vi "CAENHV Get Ch Param Prop String.vi"(6 "PropName":string, 7 "ParName":string, 8 "error in (no error)":errorcluster, 9 "Ch":u16, 10 "slot":u16, 11 "handle":i32) -> (0 "error out":errorcluster, 3 "retval":string)   [LabVIEW 2009, in "CAENHVWrapper.lvlib"]
doc: "CAENHVLIB_API CAENHVRESULT CAENHV_GetChParamProp(int handle, \n ushort slot, ushort Ch, const char *ParName, const char *PropName, void *retval);"
uses:
  <userlib>/CAENHVWrapper/CAENHVWrapper.lvlib
  <userlib>/CAENHVWrapper/CAENHVWrapper.dll
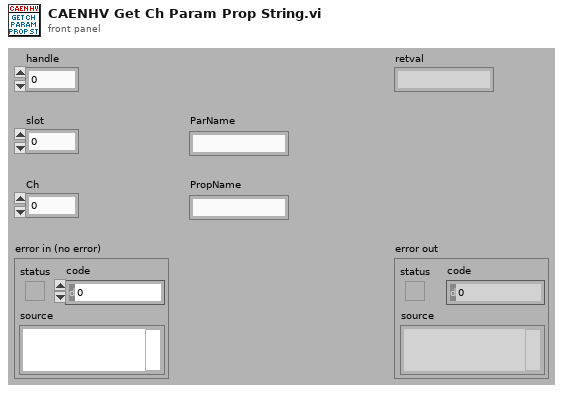
[diagram p1: front panel]
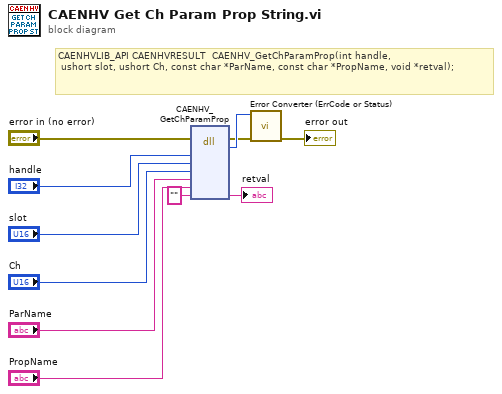
[diagram p0: block diagram]
diagram:
  # "CAENHVLIB_API CAENHVRESULT  CAENHV_GetChParamProp(int handle, \n ushort slot, ushort Ch, const char *ParName, const char *PropName, void *retval);"
  n1 = dll-call lib="C:/Program Files/National Instruments/LabVIEW 2009/user.lib/CAENHVWrapper/CAENHVWrapper.*" fn="CAENHV_GetChParamProp"(error in="error in (no error)", "handle"="handle", "slot"="slot", "Ch"="Ch", "ParName"="ParName", "PropName"="PropName", "retval"="") -> (error out=w3:errorcluster, "return type"=w4:i32, "retval"=→"retval":string)  [unwired: 7 in, 1 out]
  n2 = call <userlib>:"Error Converter (ErrCode or Status).vi"("error in (no error)"=w3, "error code"=w4) -> ("error out"=→"error out":errorcluster)  [unwired: 9 in]
